vi "CreateAllUserEvents.vi"(8 "error in (no error)":errorcluster) -> (0 "error out":errorcluster, 2 "Event Cluster":T1, 3 "Event Registration Refnum":refnum<event-registration>)   [LabVIEW 2016, in "User Events.lvlib"]
uses:
  User Events.lvlib
  controls/UI Events.ctl
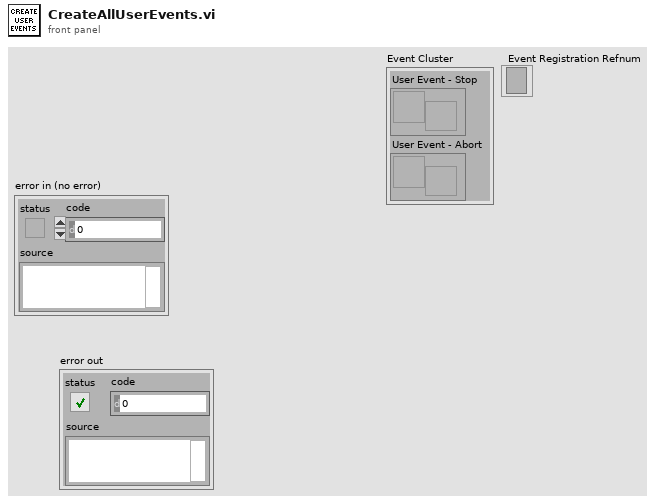
[diagram p1: front panel]
types:
  T1 = typedef "UI Events.ctl" = cluster{"User Event - Stop":refnum<user-event>, "User Event - Abort":refnum<user-event>}
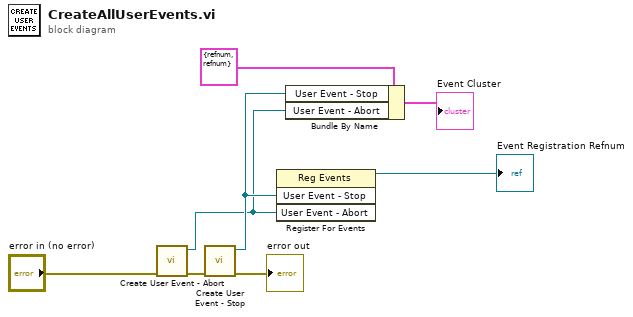
[diagram p0: block diagram]
diagram:
  n1 = call "Create User Event - Abort.vi"("error in (no error)"="error in (no error)") -> ("error out"=w4:errorcluster, "User Event - Abort"=w5:refnum<user-event>)  [unwired: 9 in]
  n2 = call "Create User Event - Stop.vi"("error in (no error)"=w4) -> ("error out"=→"error out":errorcluster, "User Event - Stop"=w7:refnum<user-event>)  [unwired: 9 in]
  n3 = register-events(w7, w5) -> (reference out=→"Event Registration Refnum":refnum<event-registration>)  [unwired: 2 in, 1 out]
  n4 = Bundle By Name(cluster=T1 {"User Event - Stop"=refnum, "User Event - Abort"=refnum} ("Event Cluster"), "User Event - Stop"=w7, "User Event - Abort"=w5) -> (→"Event Cluster":T1)
